vi "Tipo de dato boleano.vi"() -> ()   [LabVIEW 2020]
panel:
  out "Resultado OR Exclusiva":bool
  out "Resultado NOT":bool
  out "Resultado OR":bool
  out "Resultado AND":bool
  in  "Switch 3":bool
  in  "Switch 2":bool
  in  "Switch 1":bool
  in  "Boton B 9":bool
  in  "Boton B 8":bool
  in  "Boton B 7":bool
  in  "Boton B 6":bool
  in  "Boton B 5":bool
  in  "Boton B 4":bool
  in  "Boton B 3":bool
  in  "Boton B 2":bool
  out "OR":bool
  out "AND":bool
  in  "Boton B":bool
  in  "Boton A":bool
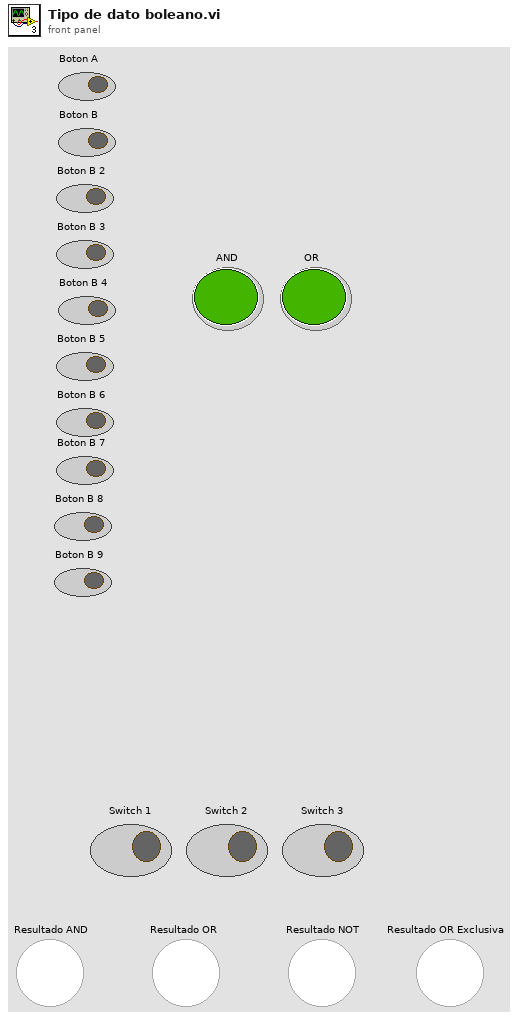
[diagram p1: front panel]
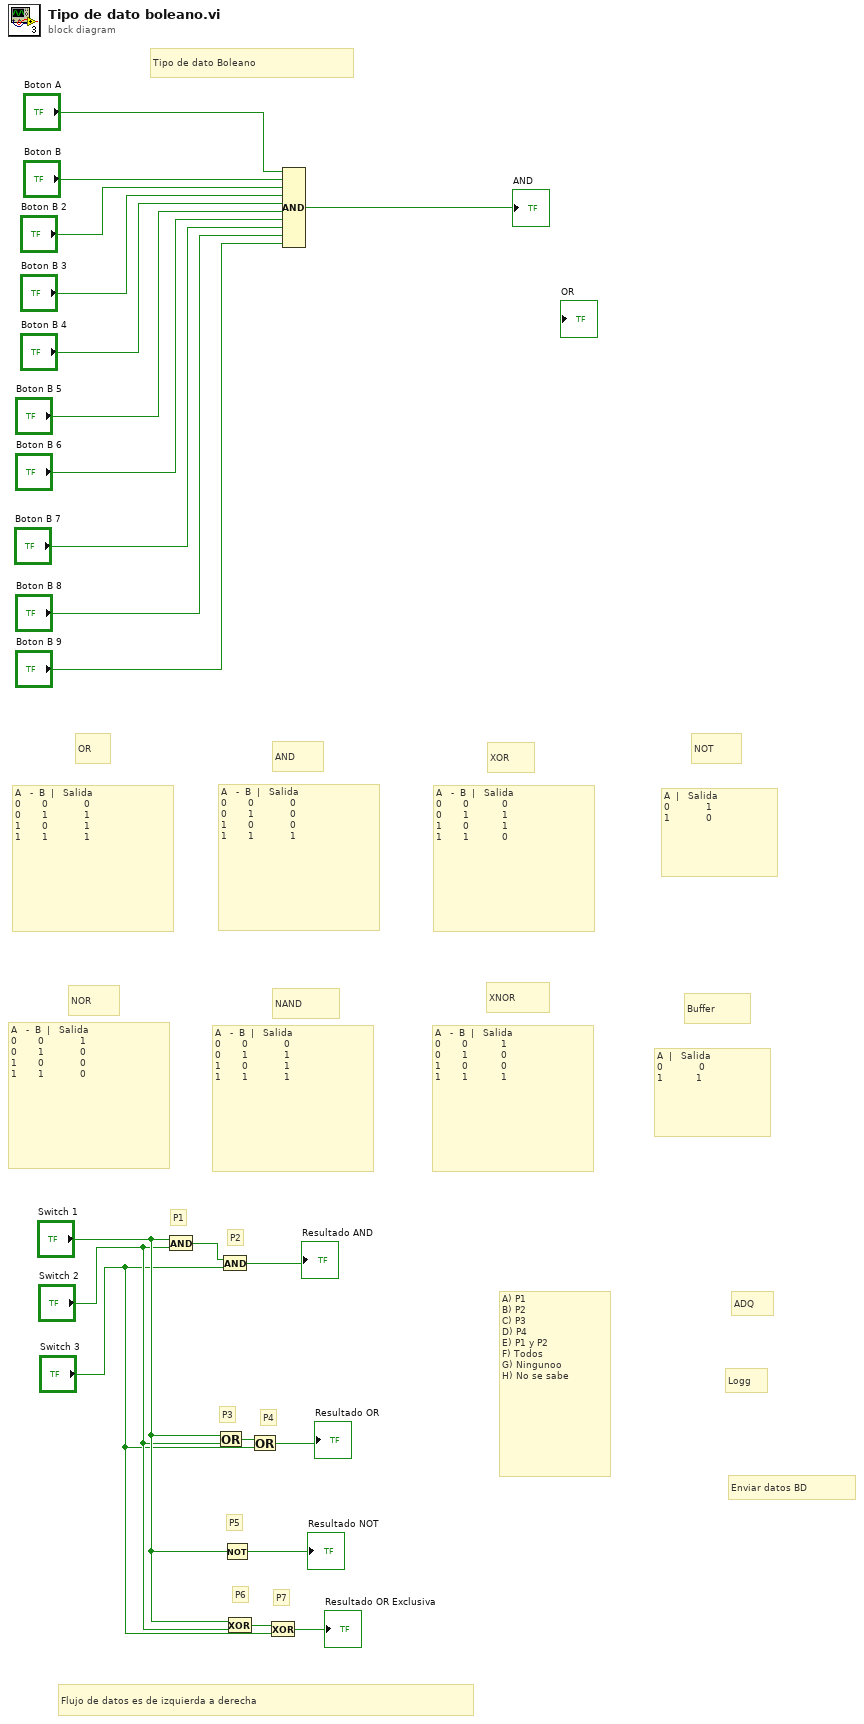
[diagram p0: block diagram]
diagram:
  # "Enviar datos BD"
  # "Logg"
  # "ADQ"
  # "Flujo de datos es de izquierda a derecha"
  # "A) P1\nB) P2\nC) P3\nD) P4\nE) P1 y P2\nF) Todos\nG) Ningunoo\nH) No se sabe"
  # "P7"
  # "P6"
  # "P5"
  # "P4"
  # "P3"
  # "P2"
  # "P1"
  # "A  |   Salida\n0            0\n1           1"
  # "Buffer"
  # "A   -  B  |   Salida\n0       0           1\n0       1           0\n1       0           0\n1       1           1"
  # "XNOR"
  # "A   -  B  |   Salida\n0       0            0\n0       1            1\n1       0            1\n1       1            1"
  # "NAND"
  # "A   -  B  |   Salida\n0       0            1\n0       1            0\n1       0            0\n1       1            0"
  # "NOR"
  # "A  |   Salida\n0            1\n1            0"
  # "NOT"
  # "A   -  B  |   Salida\n0       0           0\n0       1           1\n1       0           1\n1       1           0"
  # "XOR"
  # "A   -  B  |   Salida\n0       0            0\n0       1            0\n1       0            0\n1       1            1"
  # "A   -  B  |   Salida\n0       0            0\n0       1            1\n1       0            1\n1       1            1"
  # "AND"
  # "OR"
  # "Tipo de dato Boleano"
  n1 = And(x="Switch 1", y="Switch 2") -> (x .and. y?=w10:bool)
  n2 = Or(x="Switch 1", y="Switch 2") -> (x .or. y?=w8:bool)
  n3 = And(x=w10, y="Switch 3") -> (x .and. y?=→"Resultado AND":bool)
  n4 = Not(x="Switch 1") -> (.not. x?=→"Resultado NOT":bool)
  n5 = Exclusive Or(1:"Switch 2", 2:"Switch 1") -> (0:w3:bool)
  n6 = Or(x=w8, y="Switch 3") -> (x .or. y?=→"Resultado OR":bool)
  n7 = Exclusive Or(1:"Switch 3", 2:w3) -> (0:→"Resultado OR Exclusiva":bool)
  n8 = Compound Arithmetic op=AND("Boton A", "Boton B", "Boton B 2", "Boton B 3", "Boton B 4", "Boton B 5", "Boton B 6", "Boton B 7", "Boton B 8", "Boton B 9") -> (→"AND":bool)
